vi "getIOCdata.vi"() -> (2 "输出簇":T1)   [LabVIEW 2013]
uses:
  <userlib>/caLab/Private/Get_PV.vi
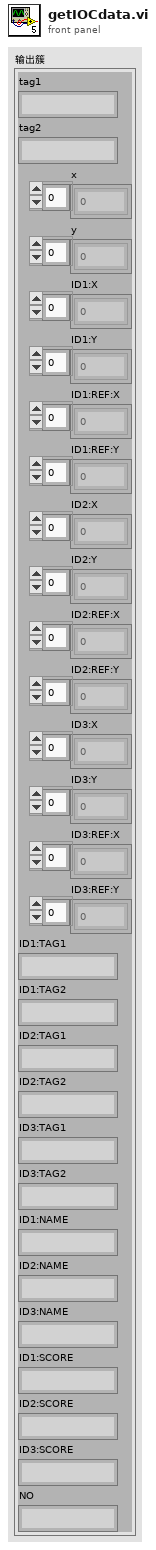
[diagram p1: front panel]
types:
  T1 = cluster{"tag1":string, "tag2":string, "x":dbl[], "y":dbl[], "ID1:X":dbl[], "ID1:Y":dbl[], "ID1:REF:X":dbl[], "ID1:REF:Y":dbl[], "ID2:X":dbl[], "ID2:Y":dbl[], "ID2:REF:X":dbl[], "ID2:REF:Y":dbl[], "ID3:X":dbl[], "ID3:Y":dbl[], "ID3:REF:X":dbl[], "ID3:REF:Y":dbl[], "ID1:TAG1":string, "ID1:TAG2":string, "ID2:TAG1":string, "ID2:TAG2":string, "ID3:TAG1":string, "ID3:TAG2":string, "ID1:NAME":string, "ID2:NAME":string, "ID3:NAME":string, "ID1:SCORE":string, "ID2:SCORE":string, "ID3:SCORE":string, "NO":string}
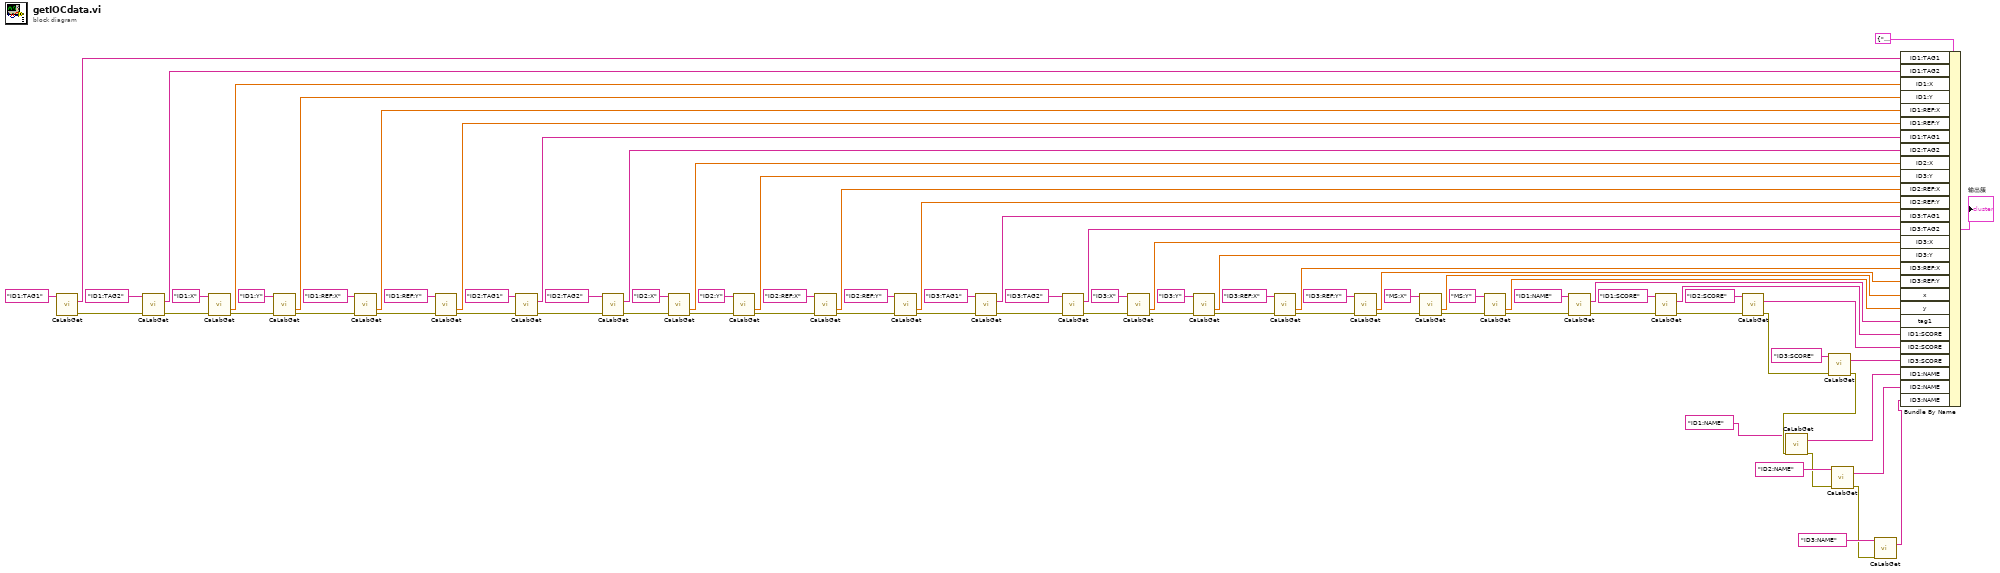
[diagram p0: block diagram]
diagram:
  n1 = call-poly <userlib>:"CaLabGet.vi"("PV Name"="ID1:TAG1") -> ("1rst Value (string)"=w81:string, "Error out"=w68:errorcluster)  [unwired: 8 in, 5 out]
  n2 = call-poly <userlib>:"CaLabGet.vi"("PV Name"="ID1:TAG2", "Error in (no error)"=w68) -> ("1rst Value (string)"=w79:string, "Error out"=w67:errorcluster)  [unwired: 7 in, 5 out]
  n3 = call-poly <userlib>:"CaLabGet.vi"("PV Name"="ID1:X", "Error in (no error)"=w67) -> ("Value Array (number)"=w77:dbl[], "Error out"=w66:errorcluster)  [unwired: 7 in, 5 out]
  n4 = call-poly <userlib>:"CaLabGet.vi"("PV Name"="ID1:Y", "Error in (no error)"=w66) -> ("Value Array (number)"=w75:dbl[], "Error out"=w65:errorcluster)  [unwired: 7 in, 5 out]
  n5 = call-poly <userlib>:"CaLabGet.vi"("PV Name"="ID1:REF:X", "Error in (no error)"=w65) -> ("Value Array (number)"=w73:dbl[], "Error out"=w64:errorcluster)  [unwired: 7 in, 5 out]
  n6 = call-poly <userlib>:"CaLabGet.vi"("PV Name"="ID1:REF:Y", "Error in (no error)"=w64) -> ("Value Array (number)"=w71:dbl[], "Error out"=w51:errorcluster)  [unwired: 7 in, 5 out]
  n7 = call-poly <userlib>:"CaLabGet.vi"("PV Name"="ID2:TAG1", "Error in (no error)"=w51) -> ("1rst Value (string)"=w39:string, "Error out"=w50:errorcluster)  [unwired: 7 in, 5 out]
  n8 = call-poly <userlib>:"CaLabGet.vi"("PV Name"="ID2:TAG2", "Error in (no error)"=w50) -> ("1rst Value (string)"=w38:string, "Error out"=w49:errorcluster)  [unwired: 7 in, 5 out]
  n9 = call-poly <userlib>:"CaLabGet.vi"("PV Name"="ID2:X", "Error in (no error)"=w49) -> ("Value Array (number)"=w37:dbl[], "Error out"=w48:errorcluster)  [unwired: 7 in, 5 out]
  n10 = call-poly <userlib>:"CaLabGet.vi"("PV Name"="ID2:Y", "Error in (no error)"=w48) -> ("Value Array (number)"=w36:dbl[], "Error out"=w47:errorcluster)  [unwired: 7 in, 5 out]
  n11 = call-poly <userlib>:"CaLabGet.vi"("PV Name"="ID2:REF:X", "Error in (no error)"=w47) -> ("Value Array (number)"=w35:dbl[], "Error out"=w46:errorcluster)  [unwired: 7 in, 5 out]
  n12 = call-poly <userlib>:"CaLabGet.vi"("PV Name"="ID2:REF:Y", "Error in (no error)"=w46) -> ("Value Array (number)"=w34:dbl[], "Error out"=w45:errorcluster)  [unwired: 7 in, 5 out]
  n13 = call-poly <userlib>:"CaLabGet.vi"("PV Name"="ID3:TAG1", "Error in (no error)"=w45) -> ("1rst Value (string)"=w33:string, "Error out"=w44:errorcluster)  [unwired: 7 in, 5 out]
  n14 = call-poly <userlib>:"CaLabGet.vi"("PV Name"="ID3:TAG2", "Error in (no error)"=w44) -> ("1rst Value (string)"=w32:string, "Error out"=w43:errorcluster)  [unwired: 7 in, 5 out]
  n15 = call-poly <userlib>:"CaLabGet.vi"("PV Name"="ID3:X", "Error in (no error)"=w43) -> ("Value Array (number)"=w31:dbl[], "Error out"=w42:errorcluster)  [unwired: 7 in, 5 out]
  n16 = call-poly <userlib>:"CaLabGet.vi"("PV Name"="ID3:Y", "Error in (no error)"=w42) -> ("Value Array (number)"=w30:dbl[], "Error out"=w41:errorcluster)  [unwired: 7 in, 5 out]
  n17 = call-poly <userlib>:"CaLabGet.vi"("PV Name"="ID3:REF:X", "Error in (no error)"=w41) -> ("Value Array (number)"=w29:dbl[], "Error out"=w40:errorcluster)  [unwired: 7 in, 5 out]
  n18 = call-poly <userlib>:"CaLabGet.vi"("PV Name"="ID3:REF:Y", "Error in (no error)"=w40) -> ("Value Array (number)"=w28:dbl[], "Error out"=w27:errorcluster)  [unwired: 7 in, 5 out]
  n19 = call-poly <userlib>:"CaLabGet.vi"("PV Name"="MS:X", "Error in (no error)"=w27) -> ("Value Array (number)"=w23:dbl[], "Error out"=w26:errorcluster)  [unwired: 7 in, 5 out]
  n20 = call-poly <userlib>:"CaLabGet.vi"("PV Name"="MS:Y", "Error in (no error)"=w26) -> ("Value Array (number)"=w22:dbl[], "Error out"=w21:errorcluster)  [unwired: 7 in, 5 out]
  n21 = call-poly <userlib>:"CaLabGet.vi"("PV Name"="ID1:NAME", "Error in (no error)"=w21) -> ("1rst Value (string)"=w19:string, "Error out"=w18:errorcluster)  [unwired: 7 in, 5 out]
  n22 = call-poly <userlib>:"CaLabGet.vi"("PV Name"="ID1:SCORE", "Error in (no error)"=w18) -> ("1rst Value (string)"=w16:string, "Error out"=w13:errorcluster)  [unwired: 7 in, 5 out]
  n23 = call-poly <userlib>:"CaLabGet.vi"("PV Name"="ID2:SCORE", "Error in (no error)"=w13) -> ("1rst Value (string)"=w14:string, "Error out"=w12:errorcluster)  [unwired: 7 in, 5 out]
  n24 = call-poly <userlib>:"CaLabGet.vi"("PV Name"="ID3:SCORE", "Error in (no error)"=w12) -> ("1rst Value (string)"=w11:string, "Error out"=w9:errorcluster)  [unwired: 7 in, 5 out]
  n25 = call-poly <userlib>:"CaLabGet.vi"("PV Name"="ID1:NAME", "Error in (no error)"=w9) -> ("1rst Value (string)"=w3:string, "Error out"=w5:errorcluster)  [unwired: 7 in, 5 out]
  n26 = call-poly <userlib>:"CaLabGet.vi"("PV Name"="ID2:NAME", "Error in (no error)"=w5) -> ("1rst Value (string)"=w2:string, "Error out"=w4:errorcluster)  [unwired: 7 in, 5 out]
  n27 = call-poly <userlib>:"CaLabGet.vi"("PV Name"="ID3:NAME", "Error in (no error)"=w4) -> ("1rst Value (string)"=w1:string)  [unwired: 7 in, 6 out]
  n28 = Bundle By Name(cluster=T1 {"tag1"="", "tag2"="", "x"=[], "y"=[], "ID1:X"=[], "ID1:Y"=[], "ID1:REF:X"=[], "ID1:REF:Y"=[], "ID2:X"=[], "ID2:Y"=[], "ID2:REF:X"=[], "ID2:REF:Y"=[], "ID3:X"=[], "ID3:Y"=[], "ID3:REF:X"=[], "ID3:REF:Y"=[], "ID1:TAG1"="", "ID1:TAG2"="", "ID2:TAG1"="", "ID2:TAG2"="", "ID3:TAG1"="", "ID3:TAG2"="", "ID1:NAME"="", "ID2:NAME"="", "ID3:NAME"="", "ID1:SCORE"="", "ID2:SCORE"="", "ID3:SCORE"="", "NO"=""}, "ID1:TAG1"=w81, "ID1:TAG2"=w79, "ID1:X"=w77, "ID1:Y"=w75, "ID1:REF:X"=w73, "ID1:REF:Y"=w71, "ID1:TAG1"=w39, "ID2:TAG2"=w38, "ID2:X"=w37, "ID3:Y"=w36, "ID2:REF:X"=w35, "ID2:REF:Y"=w34, "ID3:TAG1"=w33, "ID3:TAG2"=w32, "ID3:X"=w31, "ID3:Y"=w30, "ID3:REF:X"=w29, "ID3:REF:Y"=w28, "x"=w23, "y"=w22, "tag1"=w19, "ID1:SCORE"=w16, "ID2:SCORE"=w14, "ID3:SCORE"=w11, "ID1:NAME"=w3, "ID2:NAME"=w2, "ID3:NAME"=w1) -> (→"输出簇":T1)
